vi "libdaq_gpio_write_port.vi"(0 "error in (no error)":errorcluster, 1 "device_name":string, 2 "module_name":string, 4 "portval":bool[](array[boolean])) -> (14 "error out":errorcluster, 15 "device_name":string, 16 "module_name":string)   [LabVIEW 2010, in "libdaqVI.lvlib"]
doc: "向一个GPIO模块的所有IO写入数据，当该GPIO模块的某些IO配置为“IN”或者“AF”模式时，自动忽略对该IO的写入操作；"
uses:
  libdaqVI.lvlib
  dll/daqlib.dll
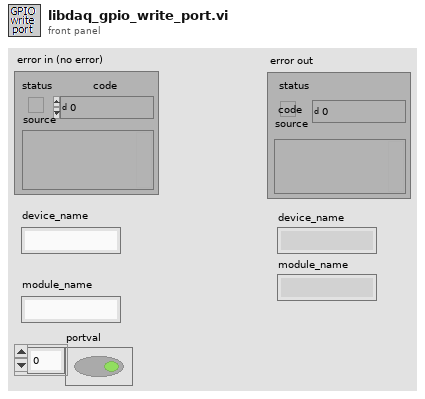
[diagram p1: front panel]
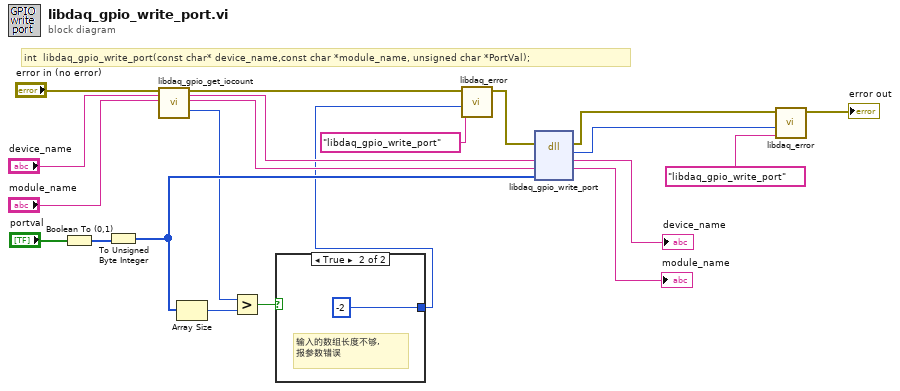
[diagram p0: block diagram]
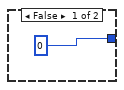
[diagram p2: hidden frame]
diagram:
  # "int  libdaq_gpio_write_port(const char* device_name,const char *module_name, unsigned char *PortVal);"
  n1 = Boolean To (0,1)(Boolean="portval") -> (0, 1=w16:i16[])
  n2 = To Unsigned Byte Integer(number=w16) -> (unsigned 8bit integer=w11:u8[])
  n3 = call "libdaq_gpio_get_iocount.vi"("error in (no error)"="error in (no error)", "device_name"="device_name", "module_name"="module_name") -> ("error out"=w3:errorcluster, "device_name"=w15:string, "module_name"=w14:string, "iocount"=w10:u8)  [unwired: 13 in]
  n4 = Array Size(array=w11) -> (size(s)=w9:i32)
  n5 = Greater?(x=w10, y=w9) -> (0:w8:bool)
  n6 = case shown="True" w8 {
    tunnel: [0 ("code") -2 ("code")] -> w6
    frame False {
    }
    frame True {
      # "输入的数组长度不够,\n报参数错误"
    }
  }
  n7 = call "libdaq_error.vi"("error source"="libdaq_gpio_write_port", "error code"=w6, "错误输入（无错误）"=w3) -> ("错误输出"=w2:errorcluster)  [unwired: 8 in]
  n8 = dll-call lib="E:/Product/Example/DAQ-USB3212/Labview/labview_2010/libdaqVI/dll/daqlib.dll" fn="libdaq_gpio_write_port"(error in=w2, "device_name"=w15, "module_name"=w14, "PortVal"=w11) -> (error out=w20:errorcluster, "return type"=w21:i32, "device_name"=→"device_name":string, "module_name"=→"module_name":string)  [unwired: 3 in, 1 out]
  n9 = call "libdaq_error.vi"("error source"="libdaq_gpio_write_port", "error code"=w21, "错误输入（无错误）"=w20) -> ("错误输出"=→"error out":errorcluster)  [unwired: 8 in]
